vi "Solve1.vi"(8 "Error In":errorcluster, 11 "object in":refnum<class "2021_14.lvclass">) -> (0 "Error Out":errorcluster, 2 "Result":u64, 3 "object out":refnum<class "2021_14.lvclass">)   [LabVIEW 2020, in "2021_14.lvclass"]
uses:
  2021_14.lvclass
  2021_14.lvclass/2021_14.ctl
  a6469d78-e4b9-4dbc-8703-66ec28e8fc39.vi
  a700af6b-bccb-4452-bcad-ec5ae36c932d.vi
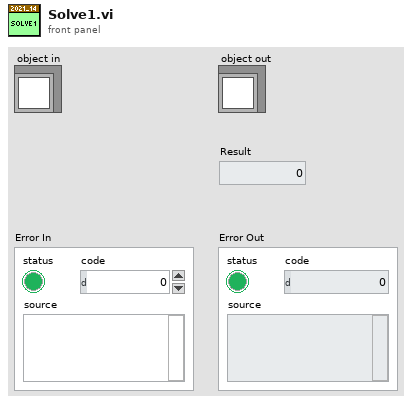
[diagram p1: front panel]
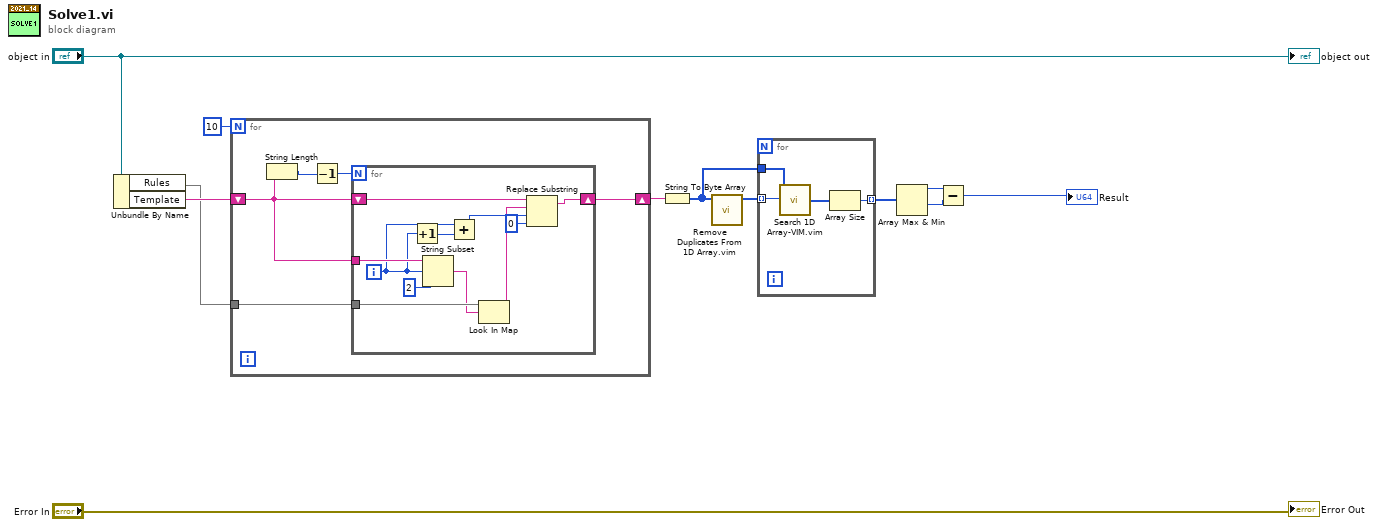
[diagram p0: block diagram]
diagram:
  n1 = Unbundle By Name("object in") -> ("Rules"=w8:map{string, string}, "Template"=w10:string)
  n2 = for {
    N: 10 -> [_]
    shift-right: [w13] -> w7
    shift-left: w10 -> [w14]
    tunnel: w8 -> [w15]
    n3 = String Length(string=w14) -> (length=w17:i32)
    n4 = Decrement(x=w17) -> (x-1=w16:i32)
    n5 = for {
      N: w16 -> [_]
      tunnel: w14 -> [w28]
      tunnel: w15 -> [w26]
      shift-right: [w23] -> w13
      shift-left: w14 -> [w24]
      i -> [w19]
      n6 = Increment(x=w19) -> (x+1=w21:i32)
      n7 = String Subset(string=w28, offset (0)=w19, length (rest)=2 ("length (rest)")) -> (substring=w25:string)
      n8 = Add(x=w19, y=w21) -> (x+y=w20:i32)
      n9 = Look In Map(map=w26, key=w25) -> (value=w22:string)  [unwired: 1 in, 1 out]
      n10 = Replace Substring(2:0 ("length (len. of substring)"), 3:w20, 4:w22, 5:w24) -> (1:w23:string)  [unwired: 1 out]
    }
  }
  n11 = String To Byte Array(string=w7) -> (unsigned byte array=w6:u8[])
  n12 = call "Remove Duplicates From 1D Array.vim"("array"=w6) -> ("array with duplicates removed"=w5:u8[])  [unwired: 10 in]
  n13 = for {
    tunnel: w6 -> [w32]
    tunnel: w5 -> [w31] mode=indexing
    tunnel: [w29] -> w4 mode=indexing
    n14 = call "Search 1D Array-VIM.vim"("Array"=w32, "Element Data"=w31) -> ("Indices of Elements"=w30:i32[])  [unwired: 7 in]
    n15 = Array Size(array=w30) -> (size(s)=w29:i32)
  }
  n16 = Array Max & Min(array=w4) -> (max value=w3:i32, min value=w2:i32)  [unwired: 2 out]
  n17 = Subtract(x=w3, y=w2) -> (x-y=→"Result":i32)
  "Error Out" <- "Error In"
  "object out" <- "object in"
